vi "Master Control.vi"(11 "Enum":T1) -> ()   [LabVIEW 2014]
uses:
  TypeDefs/SRE Enum.ctl
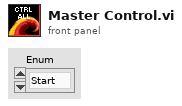
[diagram p1: front panel]
types:
  T1 = typedef "SRE Enum.ctl" = enum16{"Start", "Run", "End"}
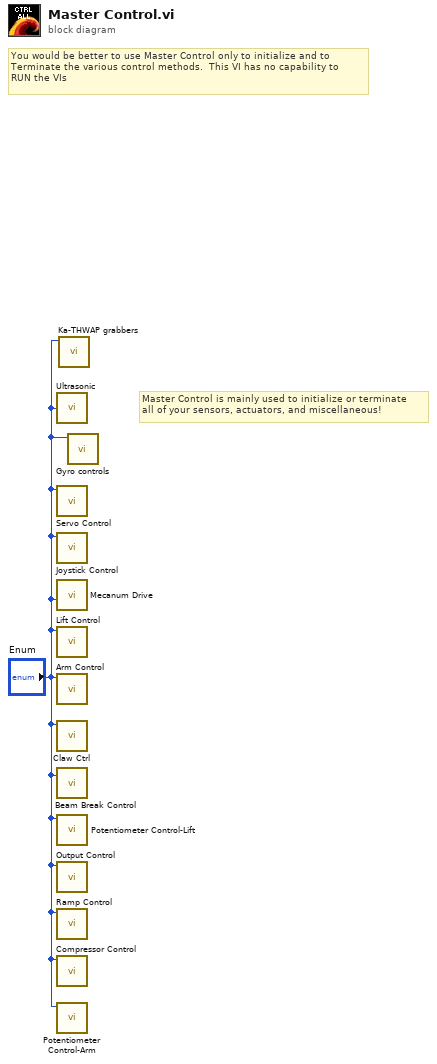
[diagram p0: block diagram]
diagram:
  # "Master Control is mainly used to initialize or terminate\nall of your sensors, actuators, and miscellaneous!"
  # "You would be better to use Master Control only to initialize and to\nTerminate the various control methods.  This VI has no capability to\nRUN the VIs"
  n1 = call "Ultrasonic.vi"("Enum"="Enum") -> ()  [unwired: 1 out]
  n2 = call "Servo Control.vi"("Enum"="Enum") -> ()  [unwired: 11 in]
  n3 = call "Joystick Control.vi"("Enum"="Enum") -> ()  [unwired: 3 in, 6 out]
  n4 = call "Mecanum Drive.vi"("Enum"="Enum") -> ()  [unwired: 11 in]
  n5 = call "Lift Control.vi"("Enum"="Enum") -> ()  [unwired: 10 in, 1 out]
  n6 = call "Arm Control.vi"("Enum"="Enum") -> ()  [unwired: 11 in]
  n7 = call "Claw Ctrl.vi"("Enum"="Enum") -> ()  [unwired: 11 in]
  n8 = call "Beam Break Control.vi"("SRE"="Enum") -> ()  [unwired: 2 in, 1 out]
  n9 = call "Potentiometer Control-Lift.vi"("Enum"="Enum") -> ()  [unwired: 10 in, 1 out]
  n10 = call "Output Control.vi"("Mode"="Enum") -> ()  [unwired: 11 in]
  n11 = call "Ramp Control.vi"("Enum"="Enum") -> ()  [unwired: 10 in]
  n12 = call "Compressor Control.vi"("Mode"="Enum") -> ()  [unwired: 11 in]
  n13 = call "Potentiometer Control-Arm.vi"("Enum"="Enum") -> ()  [unwired: 10 in, 1 out]
  n14 = call "Ka-THWAP grabbers.vi"("Enum"="Enum") -> ()  [unwired: 11 in]
  n15 = call "Gyro controls.vi"("Enum"="Enum") -> ()  [unwired: 10 in, 1 out]
